vi "Get Iteration.vi"(8 "error in (no error)":errorcluster, 10 "Iteration":i32, 11 "TTV Test in":refnum<class "Test.lvclass">) -> (0 "error out":errorcluster, 3 "TTV Test out":refnum<class "Test.lvclass">)   [LabVIEW 2019]
uses:
  Test.lvclass
  C:/Program Files (x86)/National Instruments/LabVIEW 2019/vi.lib/MGI/Panel Manager/Panel Actor/Panel Actor/Panel Actor.lvclass
  C:/Program Files (x86)/National Instruments/LabVIEW 2019/vi.lib/MGI/Monitored Actor/Monitored Actor/Monitored Actor/Monitored Actor.lvclass
  C:/Program Files (x86)/National Instruments/LabVIEW 2019/vi.lib/ActorFramework/Actor/Actor.lvclass
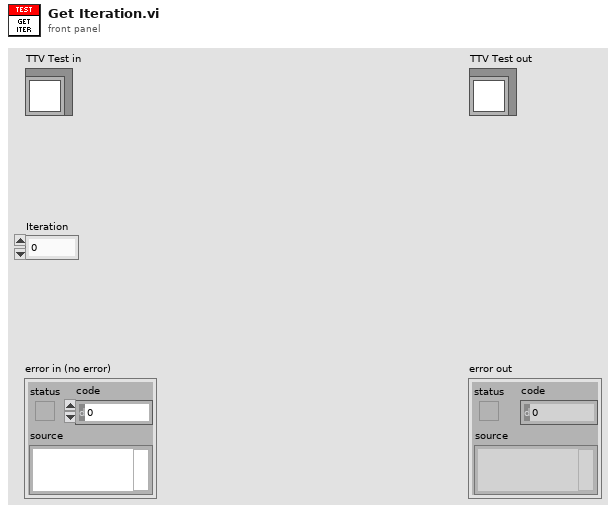
[diagram p1: front panel]
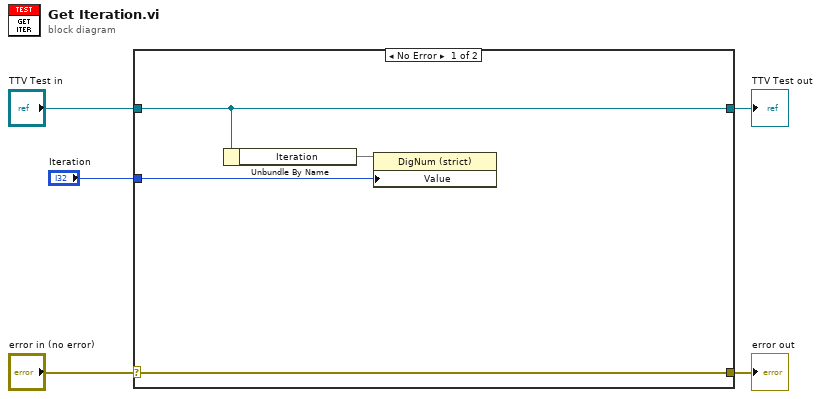
[diagram p0: block diagram]
diagram:
  n1 = case shown="No Error" "error in (no error)" {
    selector: "error in (no error)" -> [w9 w11]
    tunnel: [w9 w11] -> w4
    tunnel: [w8 w10] -> w2
    tunnel: "TTV Test in" -> [w8 w10]
    tunnel: "Iteration" -> [w6 _]
    frame No Error {
      n2 = Unbundle By Name(w8) -> ("Iteration"=w7)
      n3 = property class="DigNum (strict)"(reference=w7, "Value"=w6) -> ()  [unwired: 1 in, 2 out]
    }
    frame Error {
    }
  }
  "error out" <- w4
  "TTV Test out" <- w2
